vi "Write Ephys Task.vi"(8 "error in (no error)":errorcluster, 10 "Ephys Task":string, 11 "IntanElectrophysiology in":refnum<class "IntanElectrophysiology.lvclass">) -> (0 "error out":errorcluster, 3 "IntanElectrophysiology out":refnum<class "IntanElectrophysiology.lvclass">)   [LabVIEW 2014, in "IntanElectrophysiology.lvclass"]
uses:
  IntanElectrophysiology.lvclass
  IntanElectrophysiology.lvclass/IntanElectrophysiology.ctl
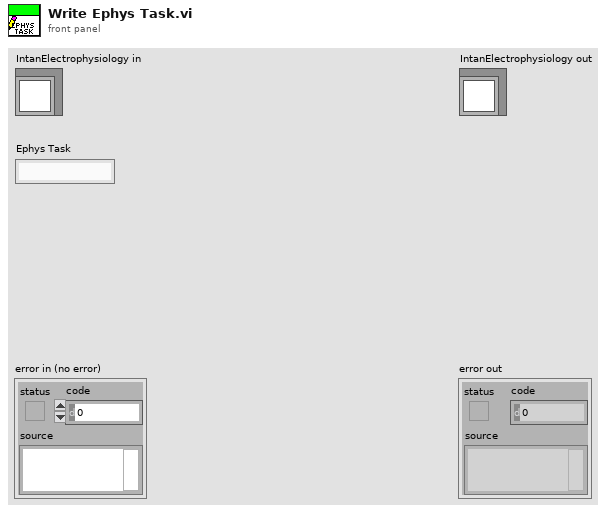
[diagram p1: front panel]
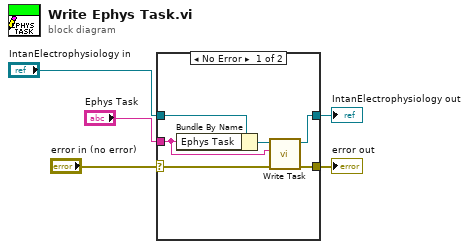
[diagram p0: block diagram]
diagram:
  n1 = case shown="No Error" "error in (no error)" {
    selector: "error in (no error)" -> [w9 w12]
    tunnel: [w8 w12] -> w4
    tunnel: [w7 w13] -> w2
    tunnel: "IntanElectrophysiology in" -> [w11 w13]
    tunnel: "Ephys Task" -> [w6 _]
    frame No Error {
      n2 = Bundle By Name(cluster=w11, "Ephys Task"=w6) -> (w10:refnum<class "IntanElectrophysiology.lvclass">)
      n3 = call-dynamic "Write Task.vi"("error in (no error)"=w9, "Task"=w6, "AcquireTraces in"=w10) -> ("error out"=w8:errorcluster, "AcquireTraces out"=w7:refnum<class "IntanElectrophysiology.lvclass">)  [unwired: 7 in]
    }
    frame Error {
    }
  }
  "error out" <- w4
  "IntanElectrophysiology out" <- w2
